vi "AMI_data.vi"() -> (0 "String":string)   [LabVIEW 2016]
uses:
  Global Variables/global.vi
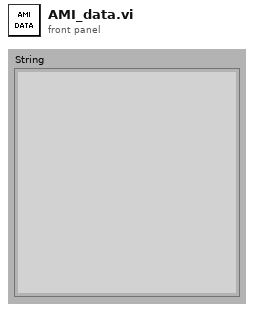
[diagram p1: front panel]
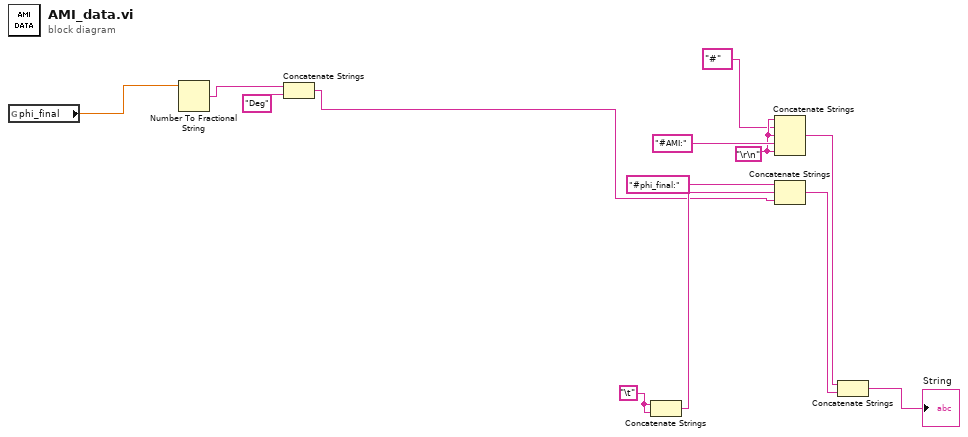
[diagram p0: block diagram]
diagram:
  w13 = "\t"
  w2 = "\r\n"
  n1 = global read "global.vi" "phi_final"() -> (w3:dbl)
  n2 = Number To Fractional String(number=w3) -> (F-format string=w5:string)  [unwired: 3 in]
  n3 = Concatenate Strings(w5, "Deg") -> (w4:string)
  n4 = Concatenate Strings(w13, w13) -> (w8:string)
  n5 = Concatenate Strings(w2, "#", w2, "#AMI:", w2) -> (w11:string)
  n6 = Concatenate Strings("#phi_final:", w8, w4) -> (w12:string)
  n7 = Concatenate Strings(w11, w12) -> (→"String":string)
